vi "Outline.vi"() -> ()   [LabVIEW 2016]
uses:
  <userlib>/LevyLab/Graph Utilities/graph_utilities.lvclass/graph_utilities.ctl
  <userlib>/LevyLab/XY Utilities/subVIs/Subset (multiple).vi
  <userlib>/LevyLab/XY Utilities/subVIs/Shift Zero (multiple).vi
  <userlib>/LevyLab/XY Utilities/subVIs/Derivative (multiple).vi
  <userlib>/LevyLab/XY Utilities/subVIs/Add float (multiple).vi
  <userlib>/LevyLab/XY Utilities/subVIs/Subset (single).vi
  <userlib>/LevyLab/XY Utilities/subVIs/Shift Zero (single).vi
  <userlib>/LevyLab/XY Utilities/subVIs/Derivative (single).vi
  <userlib>/LevyLab/XY Utilities/Swap X and Y.vi
  <userlib>/LevyLab/XY Utilities/subVIs/Swap X and Y (single).vi
  <vilib>/Analysis/2dsp.llb/Derivative x(t).vi
  <userlib>/LevyLab/XY Utilities/Private/X Array Index to Range.vi
  <vilib>/gmath/interp.llb/Interpolate 1D.vi
  <vilib>/Utility/error.llb/Error Cluster From Error Code.vi
  <userlib>/_MGI/1D Array/MGI Interpolate 1D Array Extended.vi
  <vilib>/Analysis/6fits.llb/Linear Fit.vi
  <userlib>/LevyLab/Graph Utilities/XY Graph/Set XY Graph Value (array).vi
  <userlib>/LevyLab/Graph Utilities/graph_utilities.lvclass
  <userlib>/LevyLab/XY Utilities/xy_utilities.lvlib
  <userlib>/LevyLab/LV-Data/LV-Data/LV-Data.lvclass
  <userlib>/LevyLab/LV-Data/LV-Data.ITX/LV-Data.ITX.lvclass
panel:
  in  "parameter name":string="x data"
  in  "Write Path":path=path "C:/temp"
  in  "Read Path":path=path "C:/temp"
  in  "y data name":string="y data"
  in  "x data name":string="x data"
  out "XY Graph":cluster{"Intensity Data":dbl[], "Array":dbl[]}[](graph)
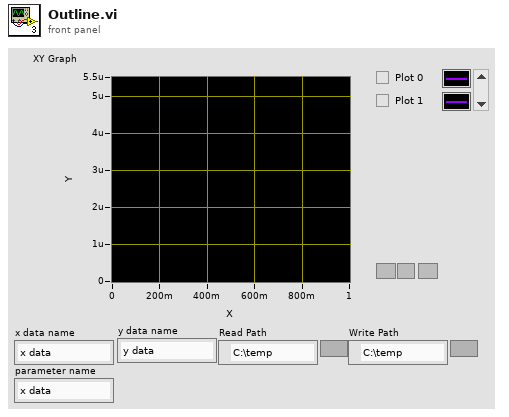
[diagram p1: front panel]
types:
  T1 = typedef "LV-Data.lvclass/Dictionary--cluster.ctl" = cluster{"key":string, "value":variant}
  T2 = typedef "Dictionary Object RefNum__ogtk.ctl" = refnum<k1>
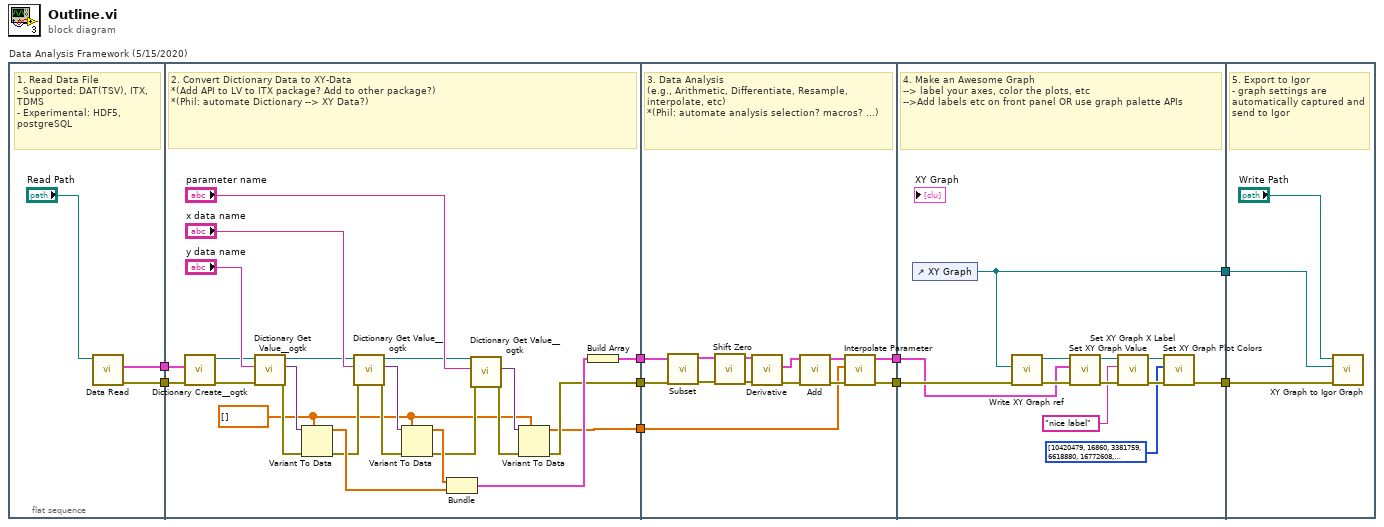
[diagram p0: block diagram]
diagram:
  n1 = flat-sequence "Data Analysis Framework (5/15/2020)" {
    tunnel: [w11] -> w9
    tunnel: [w10] -> w8
    tunnel: w9 -> [w24]
    tunnel: w8 -> [w23]
    tunnel: [w22] -> w5
    tunnel: [w16] -> w2
    tunnel: [w14] -> w1
    tunnel: [w38] -> w7
    tunnel: w5 -> [w45]
    tunnel: [w39] -> w4
    tunnel: w2 -> [w44]
    tunnel: w1 -> [w37]
    tunnel: w7 -> [w58]
    tunnel: [w57] -> w6
    tunnel: w4 -> [w53]
    tunnel: [w52] -> w3
    tunnel: w6 -> [w63]
    tunnel: w3 -> [w62]
    frame #0 {
      # "1. Read Data File\n- Supported: DAT(TSV), ITX, TDMS\n- Experimental: HDF5, postgreSQL"
      n2 = call <userlib>:"Data Read.vi"("path"="Read Path") -> ("error out"=w11:errorcluster, "Data (Dictionary)"=w10:T1[])  [unwired: 7 in, 2 out]
    }
    frame #1 {
      w15 = dbl[] []
      # "2. Convert Dictionary Data to XY-Data\n*(Add API to LV to ITX package? Add to other package?)\n*(Phil: automate Dictionary --> XY Data?)"
      n3 = call <userlib>:"Dictionary Create__ogtk.vi"("error in (no error)"=w24, "initial dictionary (empty)"=w23) -> ("error out"=w25:errorcluster, "dictionary out"=w26:T2)  [unwired: 8 in]
      n4 = call <userlib>:"Dictionary Get Value__ogtk.vi"("error in"=w25, "key"="y data name", "dictionary"=w26) -> ("error out"=w32:errorcluster, "value"=w29:variant, "dictionary out"=w27:T2)  [unwired: 5 in, 1 out]
      n5 = Variant To Data(error in=w32, type=w15, Variant=w29) -> (data=w34:dbl[], error out=w33:errorcluster)
      n6 = call <userlib>:"Dictionary Get Value__ogtk.vi"("error in"=w33, "key"="x data name", "dictionary"=w27) -> ("error out"=w35:errorcluster, "value"=w30:variant, "dictionary out"=w13:T2)  [unwired: 5 in, 1 out]
      n7 = Variant To Data(error in=w35, type=w15, Variant=w30) -> (data=w31:dbl[], error out=w18:errorcluster)
      n8 = Bundle(w31, w34) -> (w21:cluster{dbl[], dbl[]})  [unwired: 1 in]
      n9 = call <userlib>:"Dictionary Get Value__ogtk.vi"("error in"=w18, "key"="parameter name", "dictionary"=w13) -> ("error out"=w17:errorcluster, "value"=w20:variant)  [unwired: 5 in, 2 out]
      n10 = Variant To Data(error in=w17, type=w15, Variant=w20) -> (data=w14:dbl[], error out=w16:errorcluster)
      n11 = Build Array(w21) -> (w22:cluster{dbl[], dbl[]}[])
    }
    frame #2 {
      # "3. Data Analysis\n(e.g., Arithmetic, Differentiate, Resample, interpolate, etc)\n*(Phil: automate analysis selection? macros? ...)"
      n12 = call-poly <userlib>:"Subset.vi"("error in (no error)"=w44, "XY-data"=w45) -> ("error out"=w47:errorcluster, "Subset XY-data out"=w46:cluster{"X-array":dbl[], "Y-array":dbl[]}[])  [unwired: 8 in]
      n13 = call-poly <userlib>:"Shift Zero.vi"("error in (no error)"=w47, "XY-data"=w46) -> ("error out"=w42:errorcluster, "Shifted XY-data out"=w43:cluster{"X-array":dbl[], "Y-array":dbl[]}[])  [unwired: 8 in]
      n14 = call-poly <userlib>:"Derivative.vi"("error in (no error)"=w42, "XY-data"=w43) -> ("error out"=w48:errorcluster, "Differential out"=w49:cluster{"X-array":dbl[], "Y-array":dbl[]}[])  [unwired: 7 in, 1 out]
      n15 = call-poly <userlib>:"Add.vi"("error in (no error)"=w48, "XY-data"=w49) -> ("error out"=w41:errorcluster, "XY-data out"=w40:cluster{"X-array":dbl[], "Y-array":dbl[]}[])  [unwired: 8 in]
      n16 = call <userlib>:"Interpolate Parameter.vi"("error in (no error)"=w41, "Parameter-array"=w37, "XY-data"=w40) -> ("error out"=w38:errorcluster, "Interpolated XY-data out"=w39:cluster{"X-array":dbl[], "Y-array":dbl[]}[])  [unwired: 6 in, 1 out]
    }
    frame #3 {
      # "4. Make an Awesome Graph\n--> label your axes, color the plots, etc\n-->Add labels etc on front panel OR use graph palette APIs"
      n17 = control-ref of="XY Graph"() -> (w52:refnum<vi>)
      n18 = call <userlib>:"Write XY Graph ref.vi"("error in (no error)"=w58, "XY Graph"=w52) -> ("error out"=w56:errorcluster, "graph_utilities out"=w59:refnum<class "graph_utilities.lvclass">)  [unwired: 8 in]
      n19 = call-poly <userlib>:"Set XY Graph Value.vi"("error in (no error)"=w56, "XY-data"=w53, "graph_utilities in"=w59) -> ("error out"=w55:errorcluster, "graph_utilities out"=w60:refnum<class "graph_utilities.lvclass">)  [unwired: 7 in]
      n20 = call <userlib>:"Set XY Graph X Label.vi"("error in (no error)"=w55, "X Label"="nice label", "graph_utilities in"=w60) -> ("error out"=w54:errorcluster, "graph_utilities out"=w61:refnum<class "graph_utilities.lvclass">)  [unwired: 7 in]
      n21 = call <userlib>:"Set XY Graph Plot Colors.vi"("error in (no error)"=w54, "Colors []"=u32[] [10420479, 16860, 3381759, 6618880, 16772608, 16711680], "graph_utilities in"=w61) -> ("error out"=w57:errorcluster)  [unwired: 7 in, 1 out]
    }
    frame #4 {
      # "5. Export to Igor\n- graph settings are automatically captured and send to Igor"
      n22 = call <userlib>:"XY Graph to Igor Graph.vi"("error in (no error)"=w63, "XY Graph Reference"=w62, "Path"="Write Path") -> ()  [unwired: 7 in, 2 out]
    }
  }
